vi "Reset UI Colors.vi"(7 "Host":T14, 8 "error in (no error)":errorcluster, 10 "Measurement UI Controls":T17, 11 "Settings":T1) -> (0 "error out":errorcluster, 3 "Settings out":T1)   [LabVIEW 2021]
doc: "Set the colors and tooltips of UI controls back to their defaults."
uses:
  Settings/Settings.ctl
  Acquisition/Hardware Configuration.ctl
  Acquisition/Channel Settings.ctl
  Acquisition/IO Device.ctl
  Acquisition/Sensor Type.ctl
  Interval Timer/Repeat Interval.ctl
  Interval Timer/Interval Length.ctl
  Interval Timer/Interval Token.ctl
  Acquisition/IO API.ctl
  Logging/Logging Configuration.ctl
  Logging/Logging Mode.ctl
  Diagnostics/Diagnostics Configuration.ctl
  controls/Graph Settings.ctl
  controls/UI Data.ctl
  Acquisition/Host Resources.ctl
  Acquisition/Host Software Package.ctl
  Acquisition/Host IO Resource.ctl
  Settings/Settings.lvlib
  Acquisition/Acquisition.lvlib
  Interval Timer/Interval Timer.lvlib
  Logging/Logging.lvlib
  Diagnostics/Diagnostics.lvlib
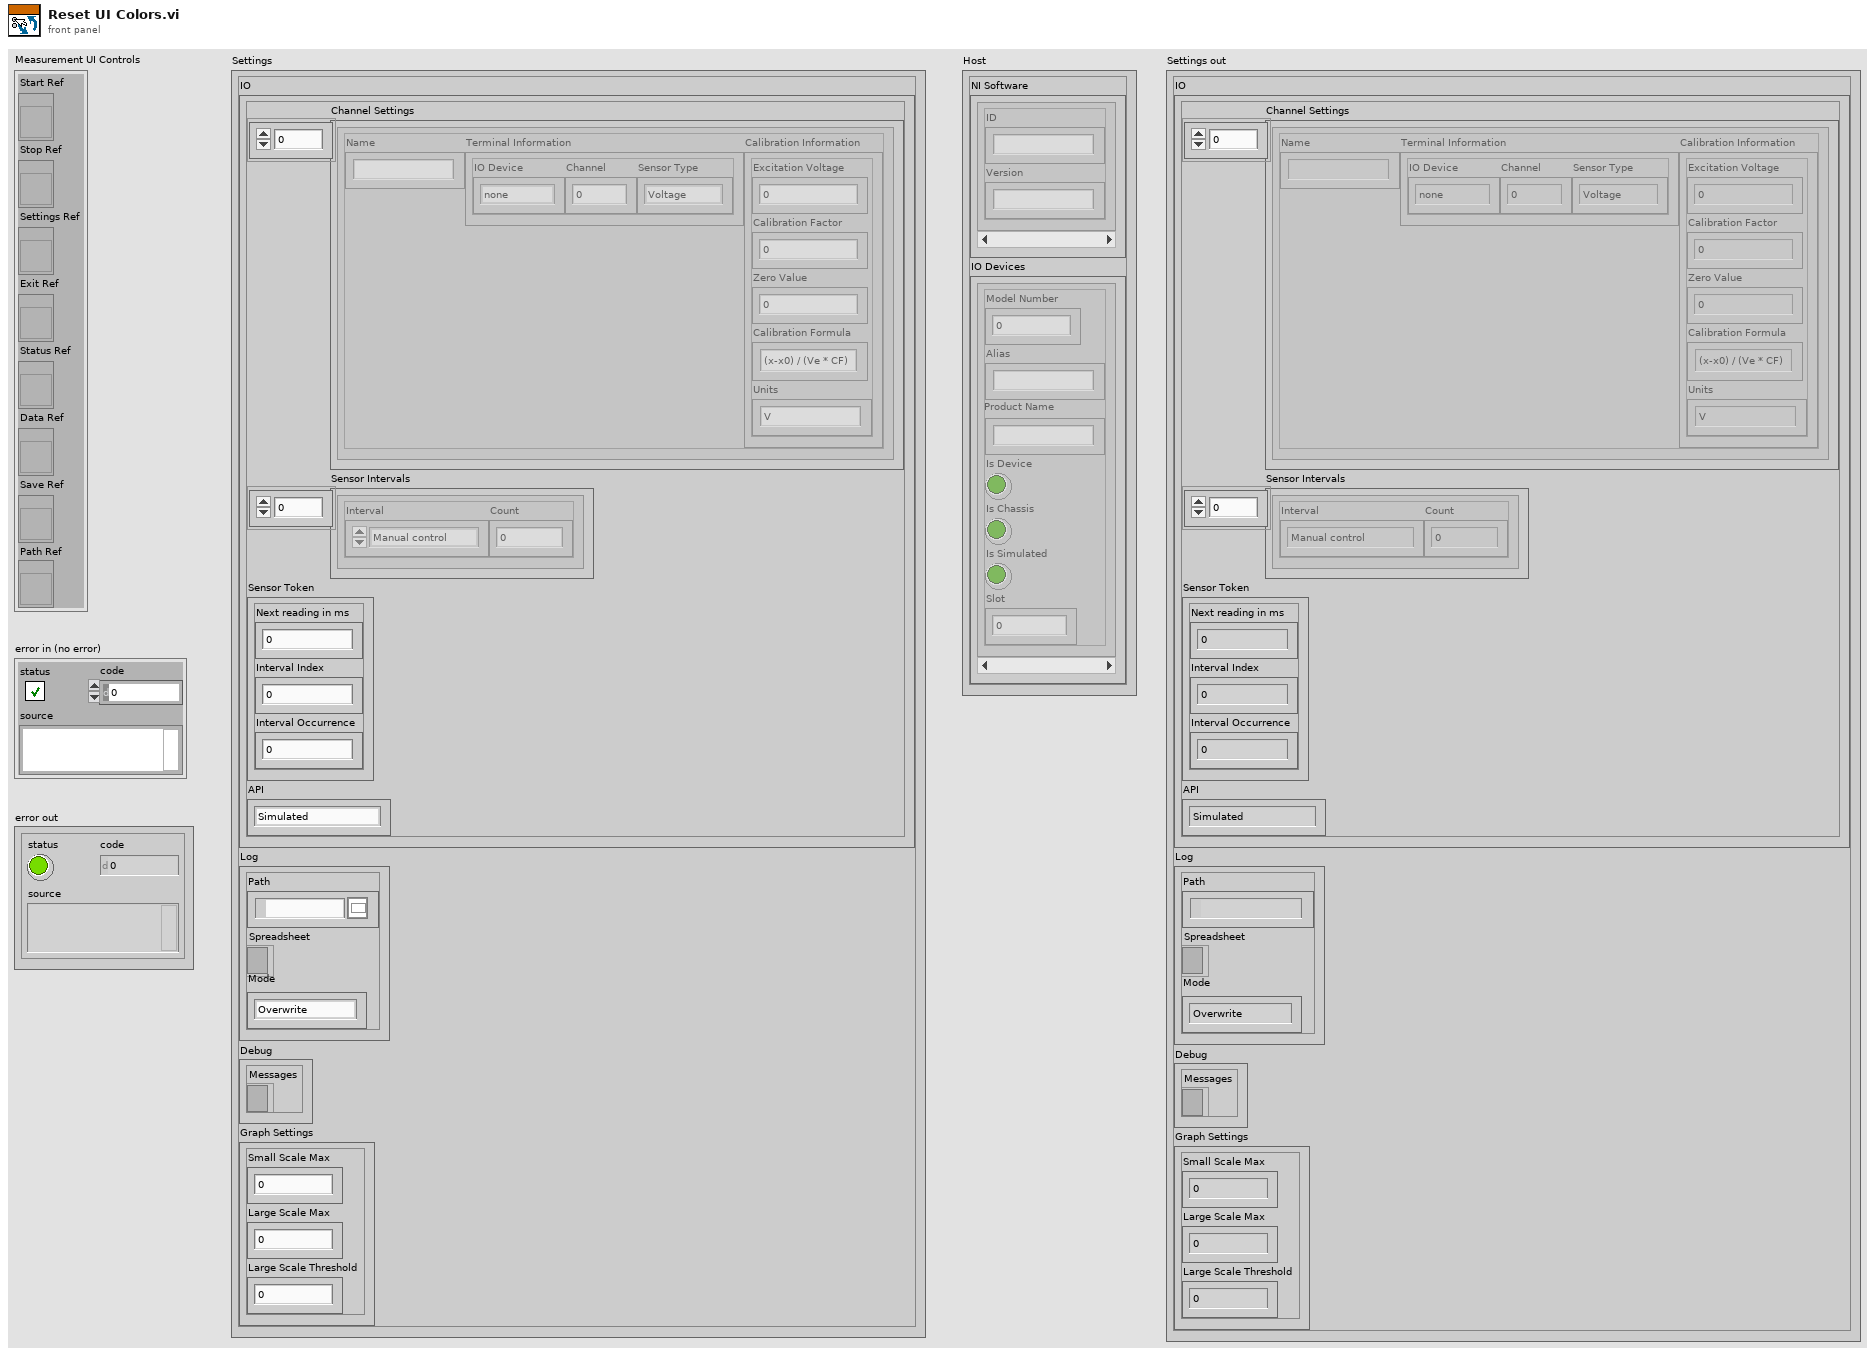
[diagram p1: front panel]
types:
  T1 = typedef "Settings.lvlib/Settings.ctl" = cluster{"IO":T2, "Log":T10, "Debug":T12, "Graph Settings":T13}
  T2 = typedef "Acquisition.lvlib/Hardware Configuration.ctl" = cluster{"Channel Settings":T3[], "Sensor Intervals":T6[], "Sensor Token":T8, "API":T9}
  T3 = typedef "Acquisition.lvlib/Channel Settings.ctl" = cluster{"Name":string, "Terminal Information":cluster{"IO Device":T4, "Channel":i32, "Sensor Type":T5}, "Calibration Information":cluster{"Excitation Voltage":dbl, "Calibration Factor":dbl, "Zero Value":dbl, "Calibration Formula":string, "Units":string}}
  T4 = typedef "Acquisition.lvlib/IO Device.ctl" = enum16{"none", "9219", "9401"}
  T5 = typedef "Acquisition.lvlib/Sensor Type.ctl" = enum16{"Voltage", "Load", "Pressure", "Encoder"}
  T6 = typedef "Interval Timer.lvlib/Repeat Interval.ctl" = cluster{"Interval":T7, "Count":i32}
  T7 = typedef "Interval Timer.lvlib/Interval Length.ctl" = enum16{"Manual control", "1 second", "10 seconds", "30 seconds", "60 seconds", "600 seconds", "1200 seconds", "3600 seconds"}
  T8 = typedef "Interval Timer.lvlib/Interval Token.ctl" = cluster{"Next reading in ms":u32, "Interval Index":i32, "Interval Occurrence":i32}
  T9 = typedef "Acquisition.lvlib/IO API.ctl" = enum16{"Simulated", "DAQmx"}
  T10 = typedef "Logging.lvlib/Logging Configuration.ctl" = cluster{"Path":path, "Spreadsheet":refnum<file>, "Mode":T11}
  T11 = typedef "Logging.lvlib/Logging Mode.ctl" = enum16{"Overwrite", "Append", "Create New"}
  T12 = typedef "Diagnostics.lvlib/Diagnostics Configuration.ctl" = cluster{"Messages":refnum<file>}
  T13 = typedef "Graph Settings.ctl" = cluster{"Small Scale Max":dbl, "Large Scale Max":dbl, "Large Scale Threshold":dbl}
  T14 = typedef "Acquisition.lvlib/Host Resources.ctl" = cluster{"NI Software":T15[], "IO Devices":T16[]}
  T15 = typedef "Acquisition.lvlib/Host Software Package.ctl" = cluster{"ID":string, "Version":string}
  T16 = typedef "Acquisition.lvlib/Host IO Resource.ctl" = cluster{"Model Number":u32, "Alias":string, "Product Name":string, "Is Device":bool, "Is Chassis":bool, "Is Simulated":bool, "Slot":i32}
  T17 = typedef "UI Data.ctl" = cluster{"Start Ref":refnum<vi>, "Stop Ref":refnum<vi>, "Settings Ref":refnum<vi>, "Exit Ref":refnum<vi>, "Status Ref":refnum<vi>, "Data Ref":refnum<vi>, "Save Ref":refnum<vi>, "Path Ref":refnum<vi>}
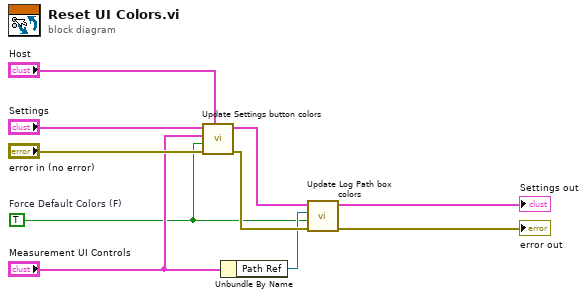
[diagram p0: block diagram]
diagram:
  w1 = TRUE  # Force Default Colors (F)
  n1 = call "Update Settings button colors.vi"("Host"="Host", "error in (no error)"="error in (no error)", "Force Default Colors (F)"=w1, "Measurement UI Controls"="Measurement UI Controls", "Settings in"="Settings") -> ("error out"=w8:errorcluster, "Settings out"=w7:T1)  [unwired: 5 in]
  n2 = Unbundle By Name("Measurement UI Controls") -> ("Path Ref"=w5:refnum<vi>)
  n3 = call "Update Log Path box colors.vi"("error in (no error)"=w8, "Force Default Colors? (F)"=w1, "Path Ref"=w5, "Settings in"=w7) -> ("error out"=→"error out":errorcluster, "Settings out"=→"Settings out":T1)  [unwired: 6 in]
